vi "PCI1240U初始化.vi"() -> (0 "DevAxesCount":u32, 1 "旋转电机":u32, 2 "电动缸电机":u32, 3 "DeviceHandle":u32, 4 "调间隙电机":u32, 5 "进给电机":u32)   [LabVIEW 2013]
panel:
  out "Device Type 2":u16(ring) items=["PCI-1220 (M0)"]
  out "AxisOpened":bool
  in  "Device Type":u16(ring) items=["PCI-1240 (M0)"]
  out "DeviceNum List":u32[](array[numeric])
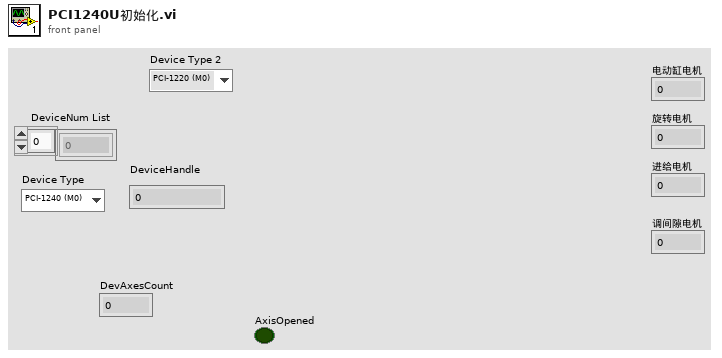
[diagram p1: front panel]
types:
  T1 = cluster{"DeviceNum":u32, "U*8 Array":cluster{"U*8 Array[0]":u8, "U*8 Array[1]":u8, "U*8 Array[2]":u8, "U*8 Array[3]":u8, "U*8 Array[4]":u8, "U*8 Array[5]":u8, "U*8 Array[6]":u8, "U*8 Array[7]":u8, "U*8 Array[8]":u8, "U*8 Array[9]":u8, "U*8 Array[10]":u8, "U*8 Array[11]":u8, "U*8 Array[12]":u8, "U*8 Array[13]":u8, "U*8 Array[14]":u8, "U*8 Array[15]":u8, "U*8 Array[16]":u8, "U*8 Array[17]":u8, "U*8 Array[18]":u8, "U*8 Array[19]":u8, "U*8 Array[20]":u8, "U*8 Array[21]":u8, "U*8 Array[22]":u8, "U*8 Array[23]":u8, "U*8 Array[24]":u8, "U*8 Array[25]":u8, "U*8 Array[26]":u8, "U*8 Array[27]":u8, "U*8 Array[28]":u8, "U*8 Array[29]":u8, "U*8 Array[30]":u8, "U*8 Array[31]":u8, "U*8 Array[32]":u8, "U*8 Array[33]":u8, "U*8 Array[34]":u8, "U*8 Array[35]":u8, "U*8 Array[36]":u8, "U*8 Array[37]":u8, "U*8 Array[38]":u8, "U*8 Array[39]":u8, "U*8 Array[40]":u8, "U*8 Array[41]":u8, "U*8 Array[42]":u8, "U*8 Array[43]":u8, "U*8 Array[44]":u8, "U*8 Array[45]":u8, "U*8 Array[46]":u8, "U*8 Array[47]":u8, "U*8 Array[48]":u8, "U*8 Array[49]":u8}, "NumOfSubDevice":i16}[]
  T2 = cluster{"U*8 Array[0]":u8, "U*8 Array[1]":u8, "U*8 Array[2]":u8, "U*8 Array[3]":u8, "U*8 Array[4]":u8, "U*8 Array[5]":u8, "U*8 Array[6]":u8, "U*8 Array[7]":u8, "U*8 Array[8]":u8, "U*8 Array[9]":u8, "U*8 Array[10]":u8, "U*8 Array[11]":u8, "U*8 Array[12]":u8, "U*8 Array[13]":u8, "U*8 Array[14]":u8, "U*8 Array[15]":u8, "U*8 Array[16]":u8, "U*8 Array[17]":u8, "U*8 Array[18]":u8, "U*8 Array[19]":u8, "U*8 Array[20]":u8, "U*8 Array[21]":u8, "U*8 Array[22]":u8, "U*8 Array[23]":u8, "U*8 Array[24]":u8, "U*8 Array[25]":u8, "U*8 Array[26]":u8, "U*8 Array[27]":u8, "U*8 Array[28]":u8, "U*8 Array[29]":u8, "U*8 Array[30]":u8, "U*8 Array[31]":u8, "U*8 Array[32]":u8, "U*8 Array[33]":u8, "U*8 Array[34]":u8, "U*8 Array[35]":u8, "U*8 Array[36]":u8, "U*8 Array[37]":u8, "U*8 Array[38]":u8, "U*8 Array[39]":u8, "U*8 Array[40]":u8, "U*8 Array[41]":u8, "U*8 Array[42]":u8, "U*8 Array[43]":u8, "U*8 Array[44]":u8, "U*8 Array[45]":u8, "U*8 Array[46]":u8, "U*8 Array[47]":u8, "U*8 Array[48]":u8, "U*8 Array[49]":u8}
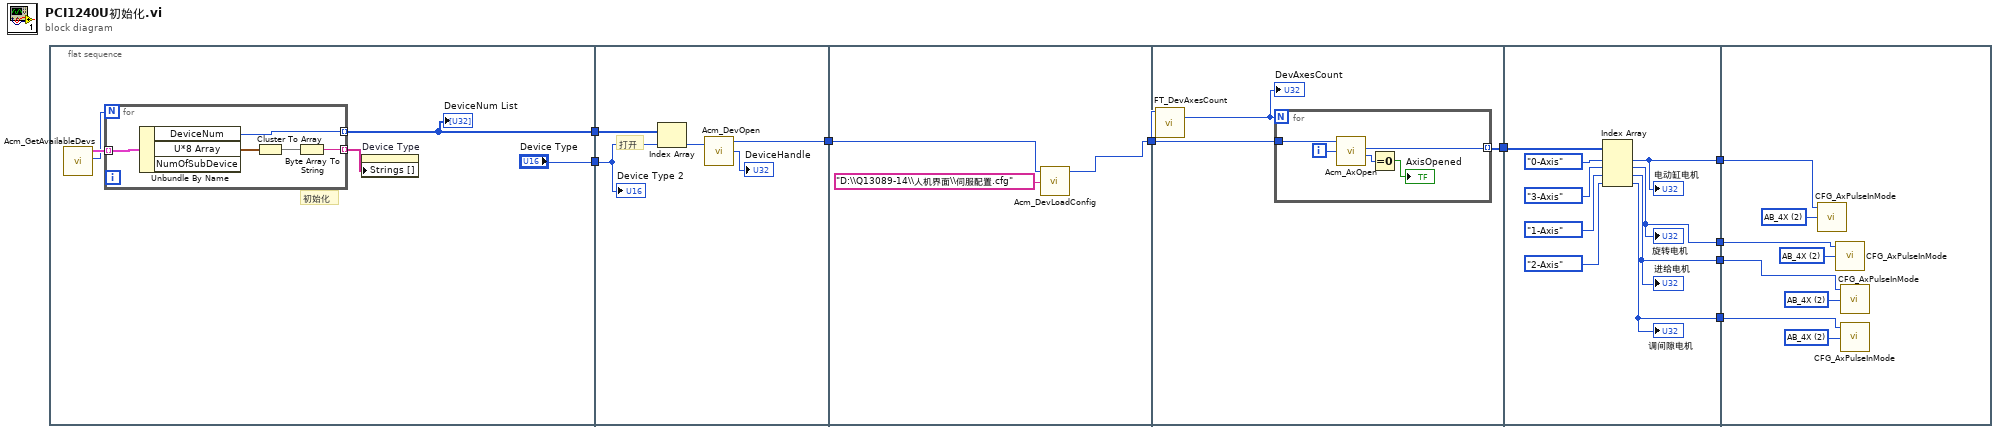
[diagram p0: block diagram]
diagram:
  n1 = flat-sequence {
    tunnel: [w13] -> w9
    tunnel: ["Device Type"] -> w8
    tunnel: w9 -> [w24]
    tunnel: w8 -> [w20]
    tunnel: [w22] -> w2
    tunnel: w2 -> [w27]
    tunnel: [w25] -> w1
    tunnel: w1 -> [w29]
    tunnel: [w28] -> w7
    tunnel: w7 -> [w44]
    tunnel: [w42] -> w6
    tunnel: [w38] -> w5
    tunnel: [w37] -> w4
    tunnel: [w36] -> w3
    tunnel: w6 -> [w45]
    tunnel: w5 -> [w48]
    tunnel: w4 -> [w47]
    tunnel: w3 -> [w46]
    frame #0 {
      # "初始化"
      n2 = call <userlib>:"Acm_GetAvailableDevs.vi"() -> ("DeviceList"=w11:T1, "OutEntries"=w10:u32)  [unwired: 3 in, 2 out]
      n3 = for {
        N: w10 -> [_]
        tunnel: w11 -> [w19] mode=indexing
        tunnel: [w16] -> w13 mode=indexing
        tunnel: [w15] -> w14 mode=indexing
        n4 = Unbundle By Name(w19) -> ("DeviceNum"=w16:u32, "U*8 Array"=w18:T2)  [unwired: 1 out]
        n5 = Cluster To Array(cluster=w18) -> (array=w17:u8[])
        n6 = Byte Array To String(unsigned byte array=w17) -> (string=w15:string)
      }
      "DeviceNum List" <- w13
      n7 = property on="Device Type" class="Ring (严格)"("Strings []"=w14) -> ()  [unwired: 2 in, 2 out]
    }
    frame #1 {
      # "打开"
      n8 = Index Array(array=w24, index=w20) -> (element=w23:u32)
      n9 = call <userlib>:"Acm_DevOpen.vi"("DeviceNumber"=w23) -> ("ReturnValue"=→"DeviceHandle":u32, "DeviceHandle"=w22:u32)  [unwired: 1 in, 1 out]
      "Device Type 2" <- w20
    }
    frame #2 {
      n10 = call <userlib>:"Acm_DevLoadConfig.vi"("ConfigPath"="D:\\Q13089-14\\人机界面\\伺服配置.cfg", "DeviceHandle"=w27) -> ("DeviceHandle"=w25:u32)  [unwired: 1 in, 2 out]
    }
    frame #3 {
      n11 = call <userlib>:"FT_DevAxesCount.vi"("Handle"=w29) -> ("DevAxesCount"=w30:u32)  [unwired: 10 in, 4 out]
      "DevAxesCount" <- w30
      n12 = for {
        N: w30 -> [_]
        tunnel: w29 -> [w35]
        tunnel: [w31] -> w28 mode=indexing
        i -> [w34]
        n13 = call <userlib>:"Acm_AxOpen.vi"("PhyAxis"=w34, "DeviceHandle"=w35) -> ("ReturnValue"=w33:u32, "AxisHandle"=w31:u32)  [unwired: 1 in, 2 out]
        n14 = Equal To 0?(x=w33) -> (x = 0?=→"AxisOpened":bool)
      }
    }
    frame #4 {
      n15 = Index Array(array=w44, index #1=enum32{"0-Axis", "1-Axis", "2-Axis", "3-Axis"}."0-Axis" ("Operate Axis"), index #2=enum32{"0-Axis", "1-Axis", "2-Axis", "3-Axis"}."3-Axis" ("Operate Axis"), index #3=enum32{"0-Axis", "1-Axis", "2-Axis", "3-Axis"}."1-Axis" ("Operate Axis"), index #4=enum32{"0-Axis", "1-Axis", "2-Axis", "3-Axis"}."2-Axis" ("Operate Axis")) -> (element #1=w42:u32, element #2=w38:u32, element #3=w37:u32, element #4=w36:u32)
      "电动缸电机" <- w42
      "旋转电机" <- w38
      "进给电机" <- w37
      "调间隙电机" <- w36
    }
    frame #5 {
      w49 = u32 2 items=["AB_1X", "AB_2X", "AB_4X", "I_CW_CCW"] ("CFG_AxPulseInMode")
      w50 = u32 2 items=["AB_1X", "AB_2X", "AB_4X", "I_CW_CCW"] ("CFG_AxPulseInMode")
      w51 = u32 2 items=["AB_1X", "AB_2X", "AB_4X", "I_CW_CCW"] ("CFG_AxPulseInMode")
      w52 = u32 2 items=["AB_1X", "AB_2X", "AB_4X", "I_CW_CCW"] ("CFG_AxPulseInMode")
      n16 = call <userlib>:"CFG_AxPulseInMode.vi"("CFG_AxPulseInMode"=w52, "Handle"=w45) -> ()  [unwired: 1 in, 3 out]
      n17 = call <userlib>:"CFG_AxPulseInMode.vi"("CFG_AxPulseInMode"=w51, "Handle"=w48) -> ()  [unwired: 1 in, 3 out]
      n18 = call <userlib>:"CFG_AxPulseInMode.vi"("CFG_AxPulseInMode"=w50, "Handle"=w47) -> ()  [unwired: 1 in, 3 out]
      n19 = call <userlib>:"CFG_AxPulseInMode.vi"("CFG_AxPulseInMode"=w49, "Handle"=w46) -> ()  [unwired: 1 in, 3 out]
    }
  }
